vi "Message type.vi"(11 "IGenericWithOutputInternalMessage in":refnum<class "IGenericWithOutputInternalMessage.lvclass">) -> (2 "Internal message type":T1, 3 "IGenericWithOutputInternalMessage out":refnum<class "IGenericWithOutputInternalMessage.lvclass">)   [LabVIEW 2020, in "wamplv.lvlib" / "IGenericWithOutputInternalMessage.lvclass"]
uses:
  IGenericWithOutputInternalMessage.lvclass
  TypeDefs/Internal message type.ctl
  wamplv.lvlib
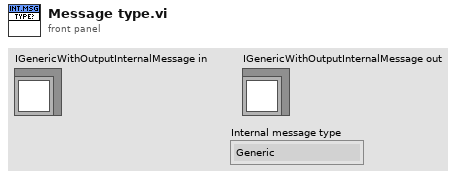
[diagram p1: front panel]
types:
  T1 = typedef "wamplv.lvlib/Internal message type.ctl" = enum16{"Generic", "Generic with write output", "Handle Result"}
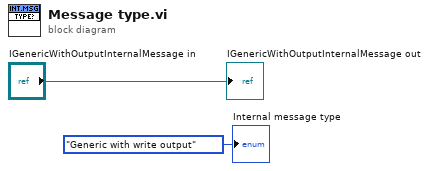
[diagram p0: block diagram]
diagram:
  "IGenericWithOutputInternalMessage out" <- "IGenericWithOutputInternalMessage in"
  "Internal message type" <- Internal_message_type."Generic with write output" ("Internal message type")
